vi "HH_SetChan.vi"(6 "error in 2":errorcluster, 7 "Dev":i32, 8 "error in":errorcluster, 10 "CHx CFD Settings":T1, 11 "Chan":i32) -> (0 "error out":errorcluster, 4 "error out 2":errorcluster)   [LabVIEW 2013]
uses:
  hhlib.dll
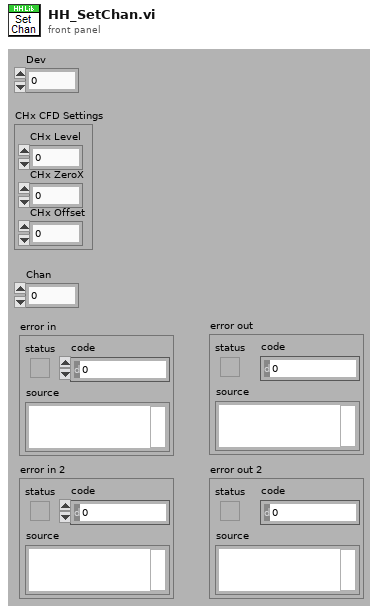
[diagram p1: front panel]
types:
  T1 = cluster{"CHx Level":i32, "CHx ZeroX":i32, "CHx Offset":i32}
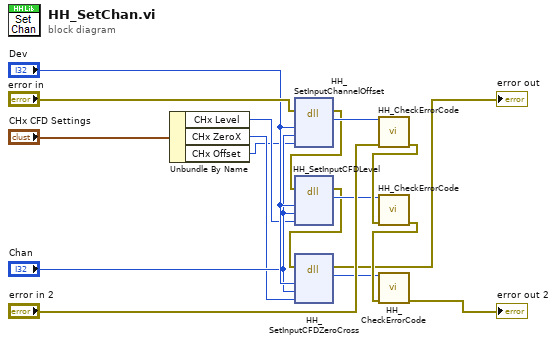
[diagram p0: block diagram]
diagram:
  n1 = Unbundle By Name("CHx CFD Settings") -> ("CHx Level"=w4:i32, "CHx ZeroX"=w3:i32, "CHx Offset"=w2:i32)
  n2 = dll-call lib="C:/Users/dhaehnel/Documents/Workspace/Labview_Workspace/labviewlib/MT Scan/SubVIs/hhlib.dll" fn="HH_SetInputChannelOffset"(error in="error in", "devidx"="Dev", "channel"="Chan", "value"=w2) -> (error out=w10:errorcluster, "return type"=w11:i32)  [unwired: 5 in, 1 out]
  n3 = dll-call lib="C:/Users/dhaehnel/Documents/Workspace/Labview_Workspace/labviewlib/MT Scan/SubVIs/hhlib.dll" fn="HH_SetInputCFDLevel"(error in=w10, "devidx"="Dev", "channel"="Chan", "value"=w4) -> (error out=w9:errorcluster, "return type"=w12:i32)  [unwired: 5 in, 1 out]
  n4 = dll-call lib="C:/Users/dhaehnel/Documents/Workspace/Labview_Workspace/labviewlib/MT Scan/SubVIs/hhlib.dll" fn="HH_SetInputCFDZeroCross"(error in=w9, "devidx"="Dev", "channel"="Chan", "value"=w3) -> (error out=→"error out":errorcluster, "return type"=w13:i32)  [unwired: 5 in, 1 out]
  n5 = call "HH_CheckErrorCode.vi"("errcode"=w11, "error in (no error)"="error in 2") -> ("error out"=w17:errorcluster)  [unwired: 12 in, 1 out]
  n6 = call "HH_CheckErrorCode.vi"("errcode"=w12, "error in (no error)"=w17) -> ("error out"=w16:errorcluster)  [unwired: 12 in, 1 out]
  n7 = call "HH_CheckErrorCode.vi"("errcode"=w13, "error in (no error)"=w16) -> ("error out"=→"error out 2":errorcluster)  [unwired: 12 in, 1 out]
